vi "All Tests.vi"(8 "error in (no error)":errorcluster) -> (0 "error out":errorcluster)   [LabVIEW 2013]
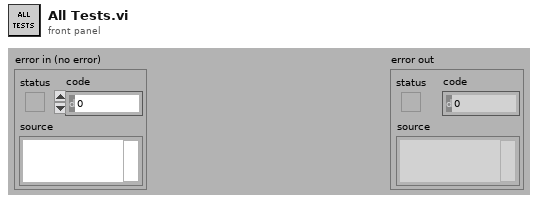
[diagram p1: front panel]
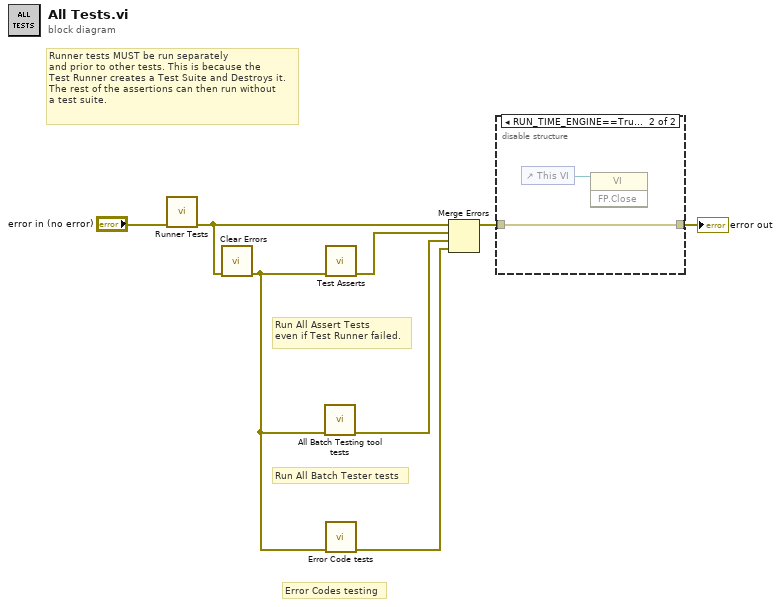
[diagram p0: block diagram]
diagram:
  # "Error Codes testing"
  # "Run All Batch Tester tests"
  # "Run All Assert Tests\neven if Test Runner failed."
  # "Runner tests MUST be run separately\nand prior to other tests. This is because the\nTest Runner creates a Test Suite and Destroys it.\nThe rest of the assertions can then run without\na test suite."
  n1 = call "Runner Tests.vi"("error in (no error)"="error in (no error)") -> ("error out"=w4:errorcluster)  [unwired: 10 in]
  n2 = call <vilib>:"Clear Errors.vi"("error in (no error)"=w4) -> ("error out"=w2:errorcluster)  [unwired: 6 in]
  n3 = call "All Batch Testing tool tests.vi"("error in (no error)"=w2) -> ("error out"=w3:errorcluster)  [unwired: 10 in]
  n4 = call "Test Asserts.vi"("error in (no error)"=w2) -> ("error out"=w6:errorcluster)  [unwired: 10 in]
  n5 = call "Error Code tests.vi"("error in (no error)"=w2) -> ("error out"=w1:errorcluster)  [unwired: 10 in]
  n6 = Merge Errors(w4, w6, w3, w1) -> (w5:errorcluster)
  n7 = disable-structure shown="RUN_TIME_ENGINE==True" {
    disable-tunnel: w5 -> [w9 w10]
    disable-tunnel: [w9 w10] -> w8
    frame condition #0 (active) {
    }
    frame condition #1 {
      n8 = control-ref of="This VI"() -> (w11:refnum<vi>)
      n9 = invoke class="VI" method="FP.Close"(reference=w11) -> ()  [unwired: 2 in, 3 out]
    }
  }
  "error out" <- w8
